vi "Set PCL Decimation_ex.vi"() -> ()   [LabVIEW 2019]
uses:
  Addon/Support Libraries/Protocols.lvlibp/Protocol Parent/Protocol Parent.lvclass
  Addon/Support Libraries/Protocols.lvlibp/Protocol Parent/Types/Base Protocol Type.ctl
  <vilib>/NI VeriStand/Custom Device API/Custom Device Item Ref.ctl
  Scripting API/Scripting API.lvlib
  <vilib>/NI VeriStand/Custom Device API/Custom Device API.lvlib
panel:
  out "instrument addon refnum out":T1=18446744073709551615 format="%.0x"
  out "error out":errorcluster
  in  "instrument addon refnum in":T1=18446744073709551615 format="%.0x"
  in  "PCL decimation":u32
  in  "error in (no error)":errorcluster
  out "protocol out":refnum<class "Protocol Parent.lvclass">
  out "protocol type":T2
  out "error out":errorcluster
  in  "protocol in":refnum<class "Protocol Parent.lvclass">
  in  "error in (no error)":errorcluster
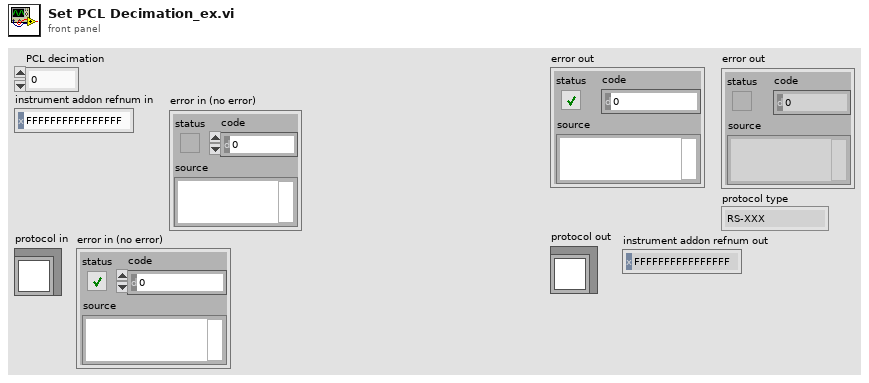
[diagram p1: front panel]
types:
  T1 = typedef "Custom Device API.lvlib/Custom Device Item Ref.ctl" = u64
  T2 = typedef "Protocols.lvlibp/Protocol Parent.lvclass/Base Protocol Type.ctl" = enum16{"RS-XXX", "VISA", "TCPIP", "UDP", "GPIB ConvBox"}
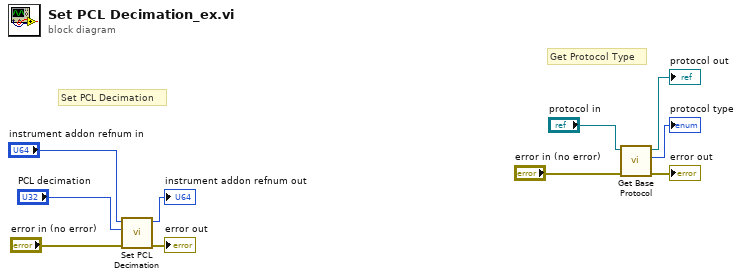
[diagram p0: block diagram]
diagram:
  # "Get Protocol Type"
  # "Set PCL Decimation"
  n1 = call "Set PCL Decimation.vi"("error in (no error)"="error in (no error)", "PCL decimation"="PCL decimation", "instrument addon refnum in"="instrument addon refnum in") -> ("error out"=→"error out":errorcluster, "instrument addon refnum out"=→"instrument addon refnum out":T1)  [unwired: 7 in]
  n2 = call-dynamic "Get Base Protocol.vi"("error in (no error)"="error in (no error)", "Protocol Parent in"="protocol in") -> ("error out"=→"error out":errorcluster, "Protocol out"=→"protocol type":T2, "Protocol Parent out"=→"protocol out":refnum<class "Protocol Parent.lvclass">)  [unwired: 7 in]
